vi "initializeTPDO.vi"(6 "error in (no error)":errorcluster, 7 "PDO channel":u8(ring) items=["PDO 1", "PDO 2", "PDO 3", "PDO 4"], 8 "interface object in":refnum<k20>, 9 "OrionBMS in":refnum<class "OrionBMSClass.lvclass">) -> (0 "error out":errorcluster, 1 "interface object out":refnum<k20>, 2 "TPDO object out":refnum<k20>, 3 "OrionBMS out":refnum<class "OrionBMSClass.lvclass">)   [LabVIEW 2018, in "OrionBMSClass.lvclass"]
uses:
  OrionBMSClass.lvclass
  <vilib>/CANopenLib/CANOPEN.llb/CANopen TPDO Create.vi
  <vilib>/CANopenLib/CANOPEN.llb/CANopen TPDO Start.vi
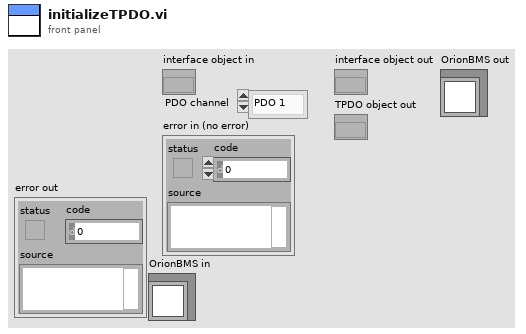
[diagram p1: front panel]
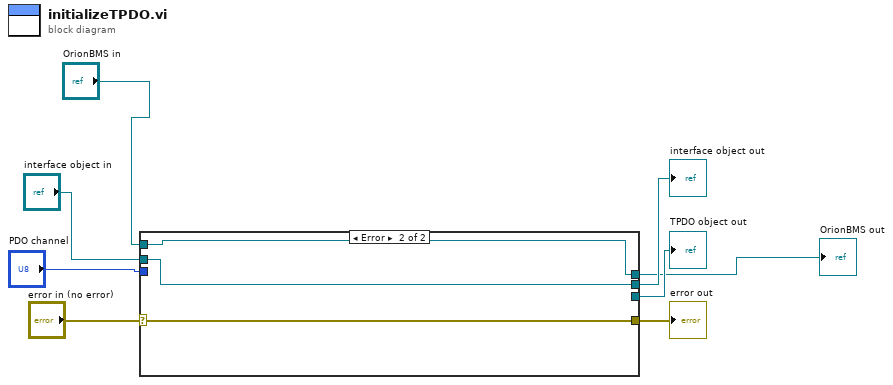
[diagram p0: block diagram]
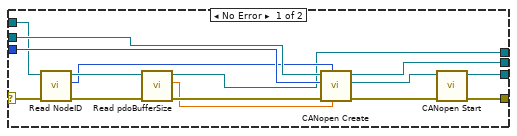
[diagram p2: hidden frame]
diagram:
  n1 = case shown="Error" "error in (no error)" {
    selector: "error in (no error)" -> [w23 w25]
    tunnel: "PDO channel" -> [w18 _]
    tunnel: "interface object in" -> [w17 w26]
    tunnel: [w14 w26] -> w5
    tunnel: [w13 _] -> w4
    tunnel: [w12 w25] -> w3
    tunnel: "OrionBMS in" -> [w10 w24]
    tunnel: [w9 w24] -> w1
    frame No Error {
      n2 = call-dynamic "Read NodeID.vi"("error in (no error)"=w23, "OrionBMS in"=w10) -> ("error out"=w22:errorcluster, "NodeID"=w15:u8, "OrionBMS out"=w19:refnum<class "OrionBMSClass.lvclass">)  [unwired: 7 in]
      n3 = call-dynamic "Read pdoBufferSize.vi"("error in (no error)"=w22, "OrionBMS in"=w19) -> ("error out"=w21:errorcluster, "pdoBufferSize"=w16:dbl, "OrionBMS out"=w9:refnum<class "OrionBMSClass.lvclass">)  [unwired: 7 in]
      n4 = call-poly <vilib>:"CANopen Create.vi"("buffer size (0)"=w16, "node-ID"=w15, "error in (no error)"=w21, "PDO channel"=w18, "interface object in"=w17) -> ("error out"=w20:errorcluster, "TPDO object out"=w11:refnum<k20>, "interface object out"=w14:refnum<k20>)  [unwired: 4 in]
      n5 = call-poly <vilib>:"CANopen Start.vi"("error in (no error)"=w20, "TPDO object in"=w11) -> ("error out"=w12:errorcluster, "TPDO object out"=w13:refnum<k20>)  [unwired: 8 in]
    }
    frame Error {
    }
  }
  "interface object out" <- w5
  "TPDO object out" <- w4
  "error out" <- w3
  "OrionBMS out" <- w1
